vi "Overwrite Item.vi"(8 "error in (no error)":errorcluster, 9 "BetterTreeItem in":refnum<class "BetterItem.lvclass">, 10 "TreeItem Index":i32, 11 "BetterBoxHandle in":refnum<class "BetterBoxHandle.lvclass">) -> (0 "error out":errorcluster, 3 "BetterBoxHandle out":refnum<class "BetterBoxHandle.lvclass">)   [LabVIEW 2020, in "BetterDragAndDrop.lvlib" / "BetterBoxHandle.lvclass"]
uses:
  BetterBoxHandle.lvclass
  C:/DSCE code/Open-source/betterdraganddrop_GIT/Source/Classes/BetterHandle/BetterHandle.lvclass
  BetterTreeItem/BetterItem.lvclass
  BetterHandle/BetterHandle.lvclass/BetterHandle.ctl
  BetterHandle/BetterHandle.lvclass
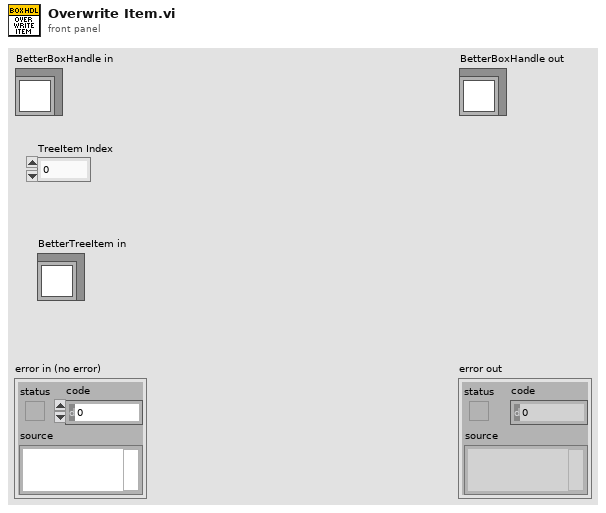
[diagram p1: front panel]
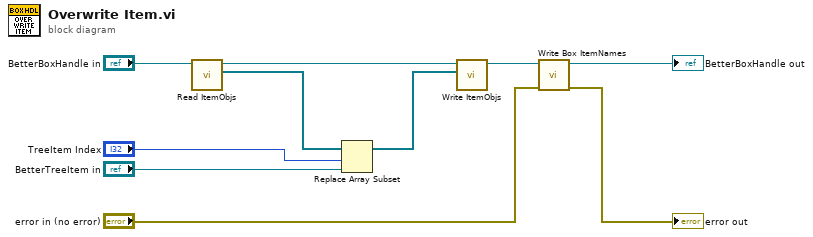
[diagram p0: block diagram]
diagram:
  n1 = call "Read ItemObjs.vi"("BetterHandle in"="BetterBoxHandle in") -> ("ItemObjs"=w7:refnum<class "BetterItem.lvclass">[], "BetterHandle out"=w10:refnum<class "BetterBoxHandle.lvclass">)  [unwired: 9 in]
  n2 = Replace Array Subset(array=w7, new element="BetterTreeItem in", index="TreeItem Index") -> (w6:refnum<class "BetterItem.lvclass">[])
  n3 = call "Write ItemObjs.vi"("ItemObjs"=w6, "BetterHandle in"=w10) -> ("BetterHandle out"=w9:refnum<class "BetterBoxHandle.lvclass">)  [unwired: 9 in]
  n4 = call-dynamic "Write Box ItemNames.vi"("error in (no error)"="error in (no error)", "BetterBoxHandle in"=w9) -> ("error out"=→"error out":errorcluster, "BetterBoxHandle out"=→"BetterBoxHandle out":refnum<class "BetterBoxHandle.lvclass">)  [unwired: 8 in]
